vi "SiosIfmWasBeamBreak.vi"(1 "Channel":i32(knob) scale=1.0..4.0, 2 "Device Number":i32) -> (0 "was broken":i32)   [LabVIEW 2009]
uses:
  siosifm.dll
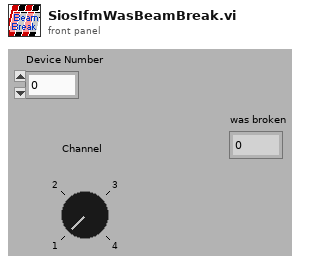
[diagram p1: front panel]
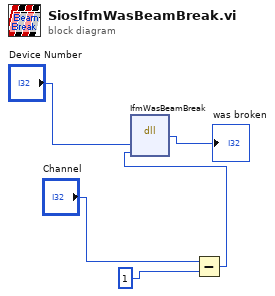
[diagram p0: block diagram]
diagram:
  n1 = Subtract(x="Channel", y=1) -> (x-y=w3:i32)
  n2 = dll-call lib="C:/WORK/Artem/RE-10/SIOS_IfmDLL/siosifm.dll" fn="IfmWasBeamBreak"("devNumber"="Device Number", "channel"=w3) -> ("was_broken"=→"was broken":i32)  [unwired: 5 in, 2 out]
